vi "Get Object Size (Channel).vi"(8 "error in (no error)":errorcluster) -> (0 "error out":errorcluster, 3 "size":u64 format="%d bytes")   [LabVIEW 2016, in "Data Sharing Framework.Runtime.lvlib"]
uses:
  Data Sharing Framework.Runtime.lvlib
  Classes/Runtime/Channel/Runtime.Channel.lvclass
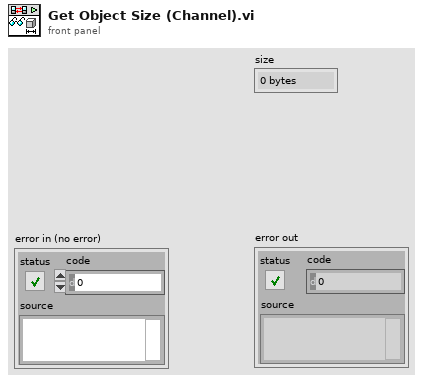
[diagram p1: front panel]
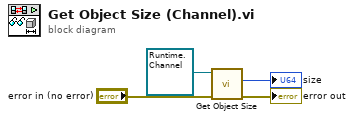
[diagram p0: block diagram]
diagram:
  n1 = call "Get Object Size.vi"("error in (no error)"="error in (no error)", "Channel Runtime in"=refnum<class "Runtime.Channel.lvclass"> refnum) -> ("error out"=→"error out":errorcluster, "size in bytes"=→"size":u64)  [unwired: 7 in, 1 out]
